vi "gearGrabber.vi"(9 "gearStatus":bool, 11 "gear":string="My Servo RefNum") -> (0 "error out":errorcluster)   [LabVIEW 2016]
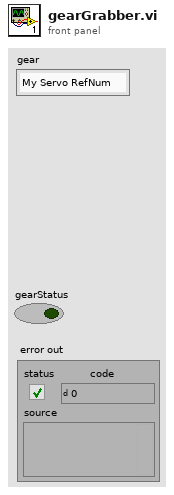
[diagram p1: front panel]
types:
  T1 = typedef "WPI_ServoDeviceRef.ctl" = cluster{"DeviceStatus":errorcluster, "PWM Channel":T2, "DeadBand":T3}
  T2 = typedef "FPGA_DIOPWMChannel.ctl" = enum8{"PWM 0", "PWM 1", "PWM 2", "PWM 3", "PWM 4", "PWM 5", "PWM 6", "PWM 7", "PWM 8", "PWM 9", "PWM MXP 0", "PWM MXP 1", "PWM MXP 2", "PWM MXP 3", "PWM MXP 4", "PWM MXP 5", "PWM MXP 6", "PWM MXP 7", "PWM MXP 8", "PWM MXP 9", "Invalid"}
  T3 = typedef "WPI_PWMDeadband.ctl" = cluster{"Name":string, "maxPositivePwm":i32, "minPositivePwm":i32, "centerPwm":i32, "maxNegativePwm":i32, "minNegativePwm":i32, "angularRange":u16}
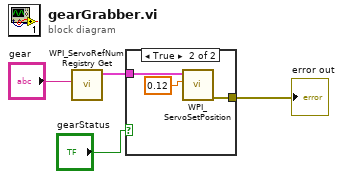
[diagram p0: block diagram]
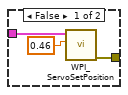
[diagram p2: hidden frame]
diagram:
  n1 = call <vilib>:"WPI_ServoRefNum Registry Get.vi"("refnum name"="gear") -> ("ServoDeviceRef"=w2:T1)  [unwired: 9 in, 1 out]
  n2 = case shown="True" "gearStatus" {
    tunnel: w2 -> [w6 w9]
    tunnel: [w5 w8] -> w1
    frame False {
      n3 = call <vilib>:"WPI_ServoSetPosition.vi"("Position"=0.46 ("gearValue"), "ServoDeviceRef"=w6) -> ("error out"=w5:errorcluster)  [unwired: 8 in, 1 out]
    }
    frame True {
      n4 = call <vilib>:"WPI_ServoSetPosition.vi"("Position"=0.12 ("gearValue"), "ServoDeviceRef"=w9) -> ("error out"=w8:errorcluster)  [unwired: 8 in, 1 out]
    }
  }
  "error out" <- w1
